vi "util_convert_version.vi"(8 "error in (no error)":errorcluster, 10 "version_delimiter":string=".", 11 "version":string) -> (0 "error out":errorcluster, 4 "build_specification_version":T1)   [LabVIEW 2015, in "lv-builder-default.lvlib"]
uses:
  lv-builder-default.lvlib
  <vilib>/AppBuilder/AB_API_Simple/Build Specification Version.ctl
  lv-build/lv-build.lvlib
  <vilib>/AppBuilder/AB_API_Simple/NI_App_Builder_API.lvlib
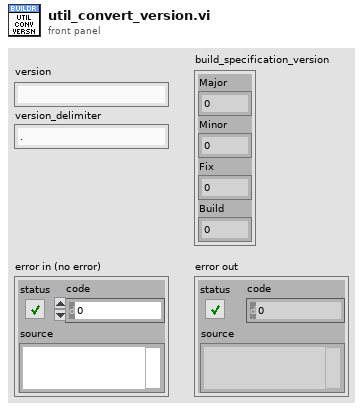
[diagram p1: front panel]
types:
  T1 = typedef "NI_App_Builder_API.lvlib/Build Specification Version.ctl" = cluster{"Major":u16, "Minor":u16, "Fix":u16, "Build":u16}
  T2 = cluster{"[0]":i32, "[1]":i32, "[2]":i32, "[3]":i32}
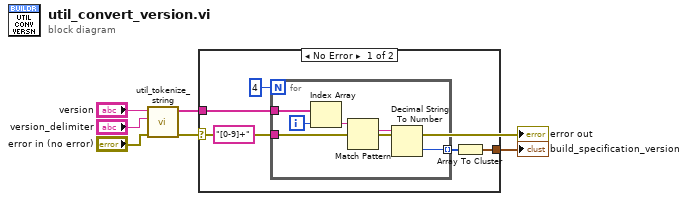
[diagram p0: block diagram]
diagram:
  n1 = call "util_tokenize_string.vi"("error in (no error)"="error in (no error)", "delimiter"="version_delimiter", "input_string"="version") -> ("error out"=w1:errorcluster, "delimited_string []"=w3:string[])  [unwired: 7 in]
  "error out" <- w1
  n2 = case shown="No Error" w1 {
    tunnel: [w9 _] -> w6
    tunnel: w3 -> [w8 _]
    frame No Error {
      n3 = for {
        N: 4 -> [_]
        tunnel: [w17] -> w10 mode=indexing
        tunnel: w8 -> [w16]
        tunnel: "[0-9]+" ("regular expression") -> [w12]
        i -> [w14]
        n4 = Index Array(array=w16, index=w14) -> (element=w15:string)
        n5 = Match Pattern(string=w15, regular expression=w12) -> (match substring=w13:string)  [unwired: 1 in, 3 out]
        n6 = Decimal String To Number(string=w13) -> (number=w17:i32)  [unwired: 2 in, 1 out]
      }
      n7 = Array To Cluster(array=w10) -> (cluster=w9:T2)
    }
    frame Error {
    }
  }
  "build_specification_version" <- w6
